vi "Msg.vi"(7 "Actor in":refnum<class "Actor.lvclass">, 11 "Terminated Msg in":refnum<class "Terminated Msg.lvclass">) -> (0 "Error out":errorcluster, 5 "Actor out":refnum<class "Actor.lvclass">)   [LabVIEW 2025, in "jettl.lvlib" / "Terminated Msg.lvlib" / "Terminated Msg.lvclass"]
uses:
  Terminated Msg.lvclass
  Terminated Msg.lvclass/Terminated Msg.ctl
  Terminated/Terminated.lvclass
  Actor/Actor/Actor.lvclass
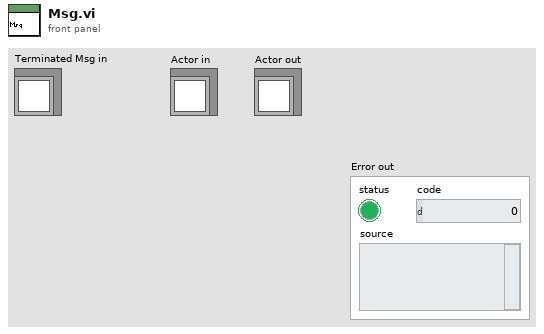
[diagram p1: front panel]
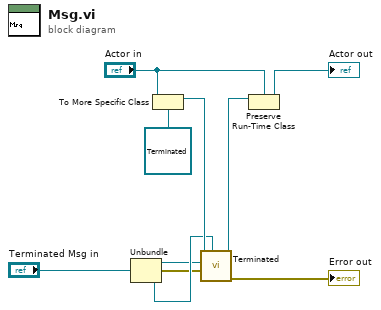
[diagram p0: block diagram]
diagram:
  n1 = Unbundle "Unbundle"("Terminated Msg in") -> (w2:refnum<class "Actor.lvclass">, w1:errorcluster, w3:refnum<class "Sender.lvclass">)
  n2 = To More Specific Class(target class=refnum<class "Terminated.lvclass"> refnum ("jettl.lvlib:jettl Msg Last Ack Creator Queue.lvlib:jettl Msg Last Ack Creator Queue.lvclass"), reference="Actor in") -> (specific class reference=w6:refnum<class "Terminated.lvclass">)  [unwired: 1 in, 1 out]
  n3 = call-dynamic "Terminated.vi"("Sender"=w3, "Error"=w1, "Actor"=w2, "Terminated in"=w6) -> ("Error out"=→"Error out":errorcluster, "Terminated out"=w5:refnum<class "Terminated.lvclass">)  [unwired: 6 in]
  n4 = Preserve Run-Time Class(object in=w5, 2:"Actor in") -> (object out=→"Actor out":refnum<class "Actor.lvclass">)  [unwired: 1 in, 1 out]
